vi "ActorNR.vi"(10 "Startup Message":refnum<class "MSG.lvclass">, 11 "Actor Type":refnum<class "Messenger.lvclass">) -> ()   [LabVIEW 2016, in "Messenger.lvclass"]
uses:
  Messenger.lvclass
  <vilib>/drjdpowell/Messenging/Core Messages/Message/MSG.lvclass
  <vilib>/drjdpowell/Messenging/ObserverRegister/ObserverRegistry.lvclass/ObserverRegistry.ctl
  <vilib>/drjdpowell/Messenging/Core Messages/Message/MSG.lvclass/MSG.ctl
  <vilib>/drjdpowell/Messenging/Core Messages/ErrorMessage/ErrorMSG.lvclass/ErrorMSG.ctl
  <vilib>/Utility/error.llb/DialogType.ctl
  <vilib>/drjdpowell/Messenging/Core Messages/ErrorMessage/Write ErrorMessage.vi
  <vilib>/drjdpowell/Messenging/Core Messages/MSG Library/Reply (message).vi
  <vilib>/drjdpowell/Messenging/Core Messages/MSG Library/Reply (no data).vi
  <vilib>/drjdpowell/Messenging/Core Messages/Message/Label Message.vi
  <vilib>/drjdpowell/Messenging/ObserverRegister/Read DVR.vi
  <vilib>/drjdpowell/Messenging/Core Messages/Message/Write (no data).vi
  <vilib>/drjdpowell/Messenging/Core Messages/Message/Overwrite Reply Address.vi
  <vilib>/drjdpowell/Messenging/Core Messages/ErrorMessage/ErrorMSG.lvclass
  C:/Program Files (x86)/National Instruments/LabVIEW 2016/vi.lib/drjdpowell/Messenging/Core Messages/Message/MSG.lvclass
  <vilib>/drjdpowell/Messenging/ObserverRegister/ObsReg Core/Event Notification.vi
  <vilib>/drjdpowell/Messenging/ObserverRegister/Commands/ParentCommand/ObserverRegistryCommand.lvclass
  <vilib>/drjdpowell/Messenging/Core Messengers/Send/Send.lvclass
  <vilib>/drjdpowell/Messenging/Core Messengers/EventMessenger/EventMessenger.lvclass
  <vilib>/drjdpowell/Messenging/Core Messages/MSG Library/SendMSG.lvlib
  <vilib>/drjdpowell/Messenging/ObserverRegister/ObsReg.lvlib
  <vilib>/drjdpowell/Messenging/Parallel Process/Parallel Process Library/Parallel Process.lvlib
  <vilib>/drjdpowell/Messenging/ObserverRegister/ObserverRegistry.lvclass
panel:
  # "You can make this actor shared-reentrant (many instances)\nor non-reentrant (only one instance).\nTo do so you must also rename this VI:\n     shared reentrant: \"Actor.vi\"\n     non-reentrant: \"ActorNR.vi\""
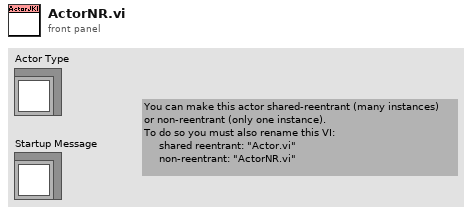
[diagram p1: front panel]
types:
  T1 = typedef "Parallel Process.lvlib/Actor Communication.ctl" = cluster{"Messenger":refnum<class "EventMessenger.lvclass">, "Private Messenger":refnum<class "EventMessenger.lvclass">, "ObsReg":refnum<class "ObserverRegistry.lvclass">, "Reg":refnum<event-registration>}
  T2 = enum32{"invalid app kind", "Development System", "Run Time System", "Student Edition", "Embedded LabVIEW", "Evaluation", "Custom"}
  T3 = enum32{"Invalid", "Standard", "Closed", "Hidden", "Minimized", "Maximized"}
  T4 = cluster{"Core":cluster{"Current VI Reference":refnum<vi>, "Close Panel on Exit?":bool, "Running Top Level":bool}, "Actor":T1, "Your Boolean data":bool, "TimeFormat":string}
  T5 = typedef "DialogType.ctl" = u16
  T6 = enum16{"Left Button", "Center Button", "Right Button", "Window Close"}
  T7 = cluster{"Current VI Reference":refnum<vi>, "Close Panel on Exit?":bool, "Running Top Level":bool}
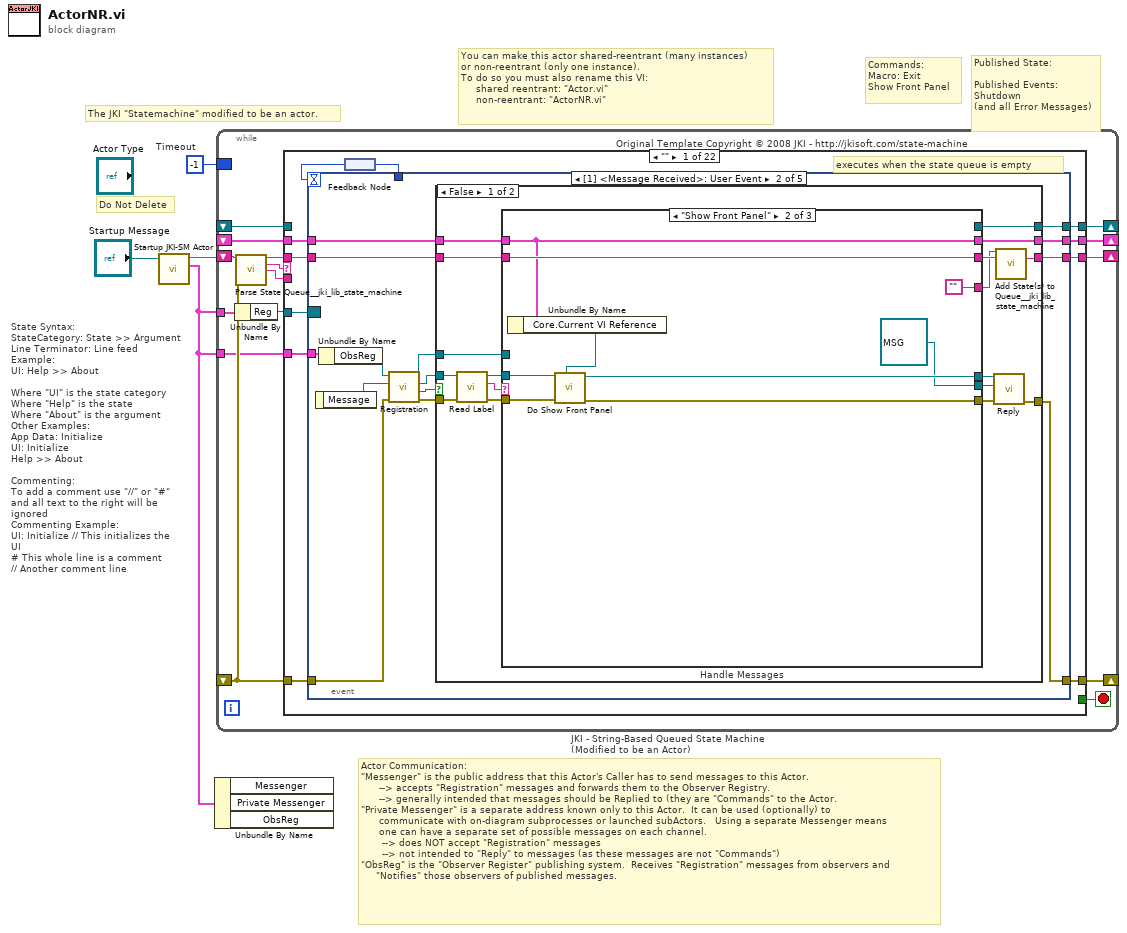
[diagram p0: block diagram]
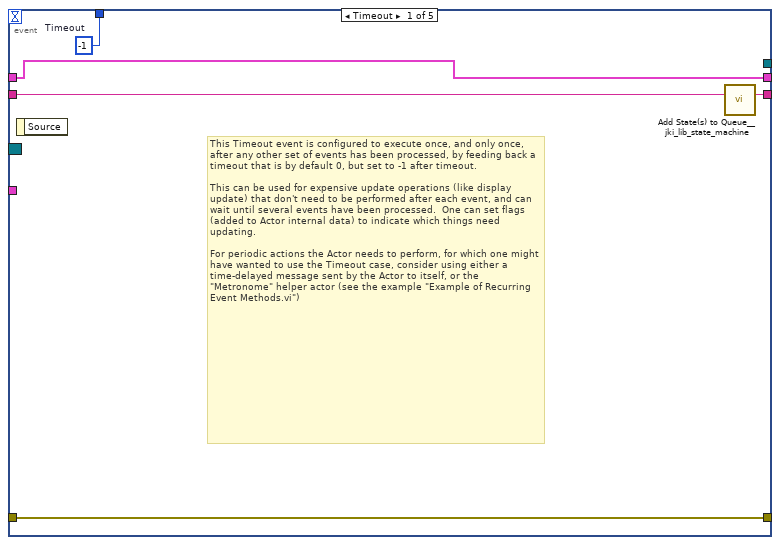
[diagram p2: hidden frame]
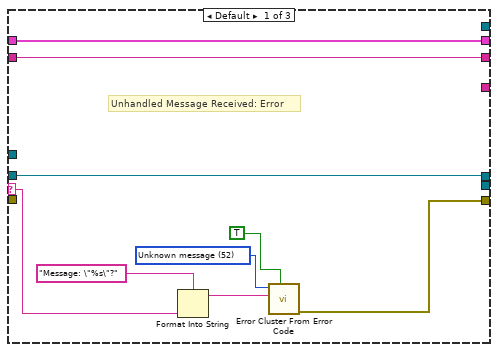
[diagram p3: hidden frame]
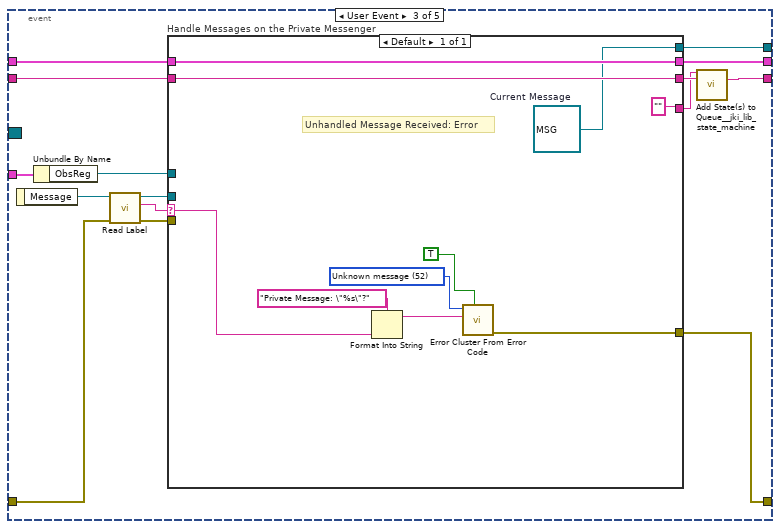
[diagram p6: hidden frame]
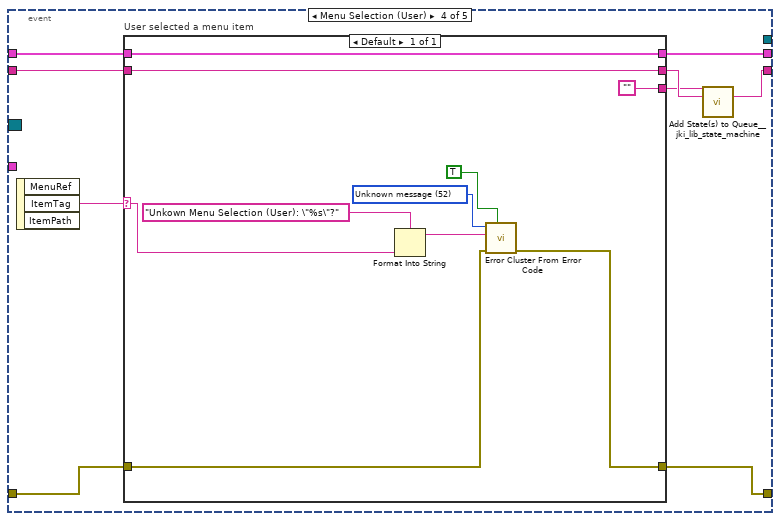
[diagram p7: hidden frame]
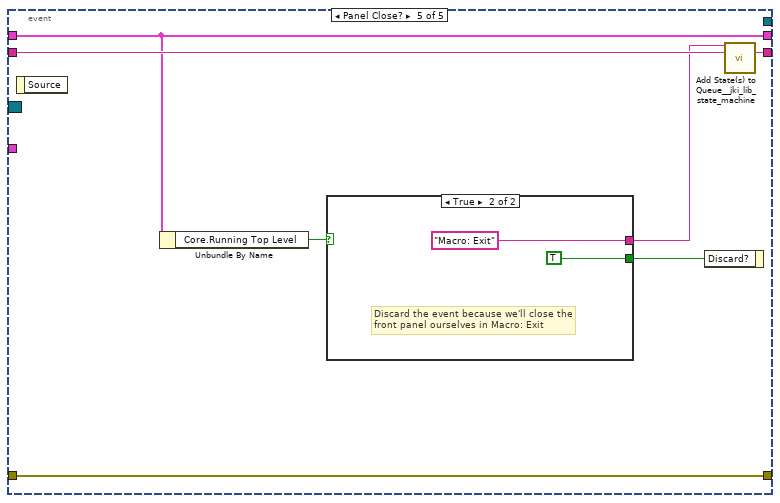
[diagram p8: hidden frame]
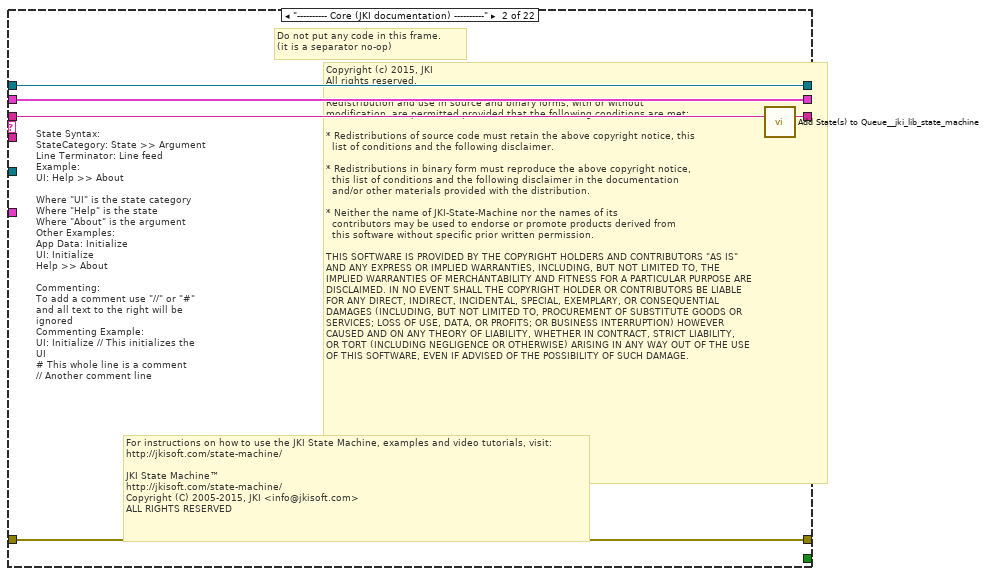
[diagram p10: hidden frame]
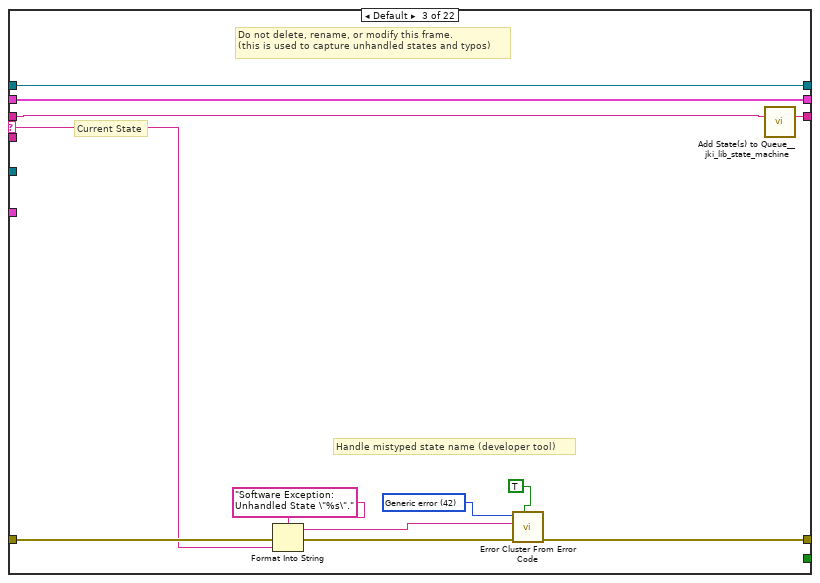
[diagram p11: hidden frame]
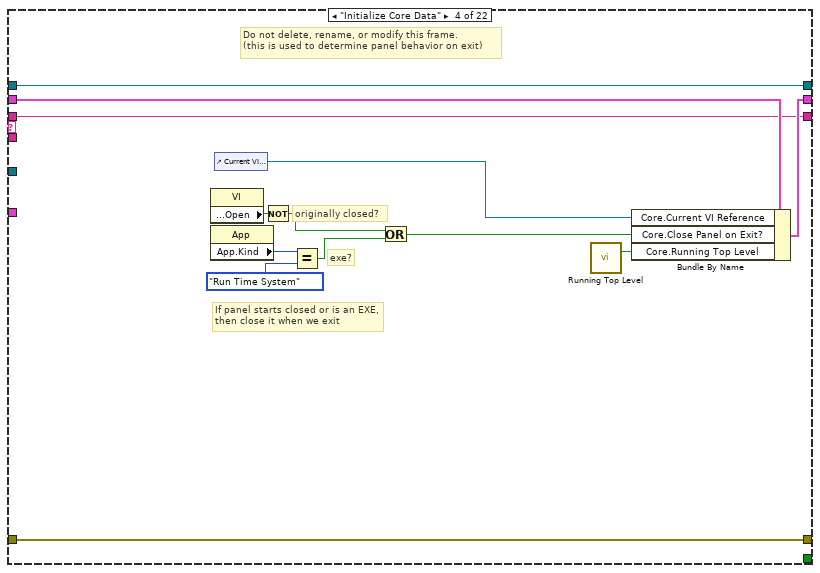
[diagram p12: hidden frame]
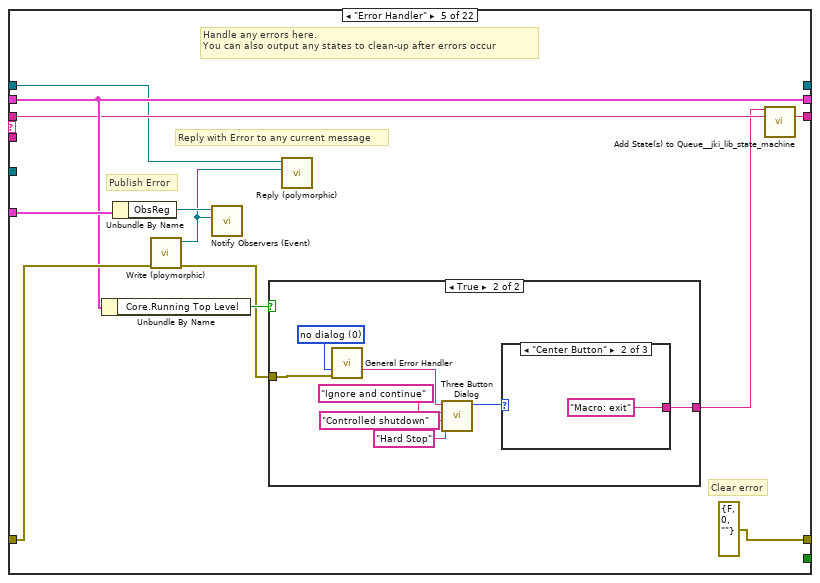
[diagram p13: hidden frame]
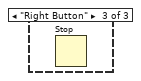
[diagram p16: hidden frame]
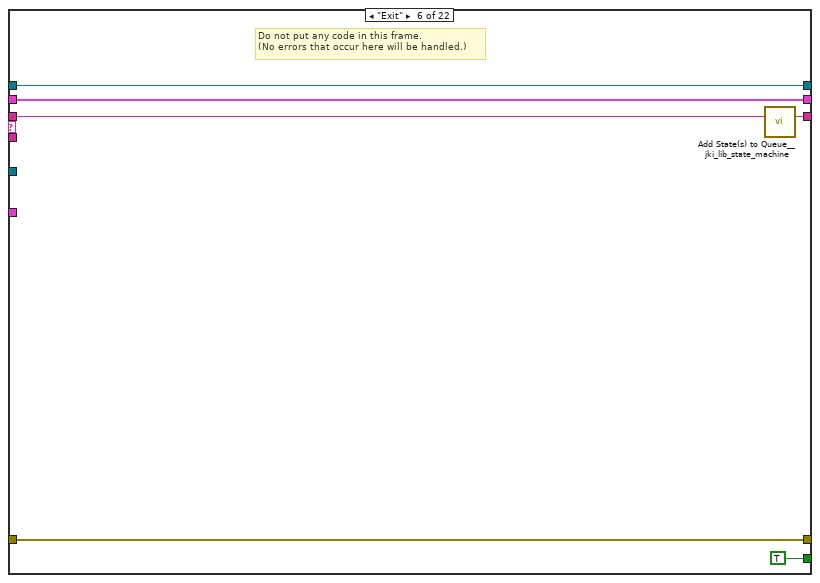
[diagram p17: hidden frame]
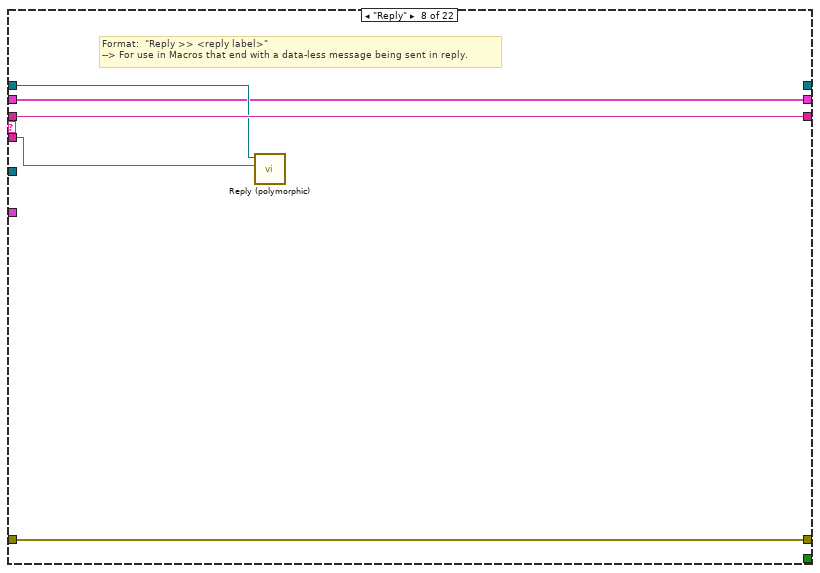
[diagram p19: hidden frame]
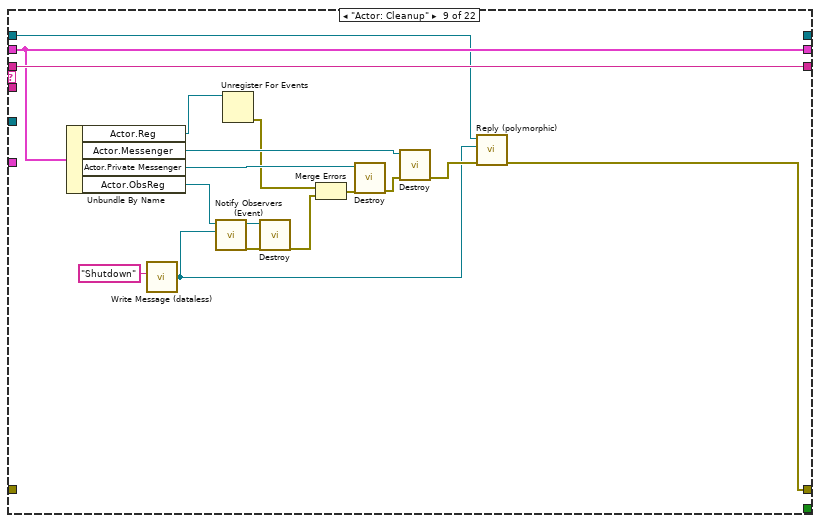
[diagram p20: hidden frame]
diagram:
  w1 = -1  # Timeout
  # "You can make this actor shared-reentrant (many instances)\nor non-reentrant (only one instance).\nTo do so you must also rename this VI:\n     shared reentrant: \"Actor.vi\"\n     non-reentrant: \"ActorNR.vi\""
  # "State Syntax:\nStateCategory: State >> Argument\nLine Terminator: Line feed\nExample:\nUI: Help >> About\n\nWhere \"UI\" is the state category\nWhere \"Help\" is the state\nWhere \"About\" is the argument\nOther Examples:\nApp Data: Initialize\nUI: Initialize\nHelp >> About\n\nCommenting:\nTo add a comment use \"//\" or \"#\" and all text to the right will be ignored\nCommenting Example:\nUI: Initialize // This initializes the UI\n# This whole line is a comment\n// Another comment line"
  # "The JKI \"Statemachine\" modified to be an actor."
  # "Actor Communication:\n\"Messenger\" is the public address that this Actor's Caller has to send messages to this Actor.\n      --> accepts \"Registration\" messages and forwards them to the Observer Registry.\n      --> generally intended that messages should be Replied to (they are \"Commands\" to the Actor.\n\"Private Messenger\" is a separate address known only to this Actor.  It can be used (optionally) to \n      communicate with on-diagram subprocesses or launched subActors.   Using a separate Messenger means\n      one can have a separate set of possible messages on each channel. \n       --> does NOT accept \"Registration\" messages\n       --> not intended to \"Reply\" to messages (as these messages are not \"Commands\")\n\"ObsReg\" is the \"Observer Register\" publishing system.  Receives \"Registration\" messages from observers and \n     \"Notifies\" those observers of published messages."
  # "Do Not Delete"
  # "Published State:\n \nPublished Events:\nShutdown\n(and all Error Messages)"
  # "Commands:\nMacro: Exit\nShow Front Panel"
  n1 = call <vilib>:"Startup JKI-SM Actor.vi"("MSG in"="Startup Message") -> ("Actor"=w2:T1, "Initial States (\"Macro: Initialize\")"=w3:string)  [unwired: 9 in]
  n2 = Unbundle By Name(w2) -> ()  [unwired: 3 out]
  n3 = while "JKI - String-Based Queued State Machine (Modified to be an Actor)" {
    shift-right: [w12] -> _
    shift-left: _ -> [w11]
    shift-right: [w15] -> _
    shift-left: _ -> [w10]
    shift-right: [w14] -> _
    shift-left: w3 -> [w16]
    tunnel: w2 -> [w7]
    tunnel: w2 -> [w9]
    shift-right: [w6] -> _
    shift-left: _ -> [w5]
    border: w1 -> [_]
    stop <- w13 stop-if-true
    # "Original Template Copyright © 2008 JKI - http://jkisoft.com/state-machine"
    n4 = Unbundle By Name(w7) -> ("Reg"=w8:refnum<event-registration>)
    n5 = call <vilib>:"Parse State Queue__jki_lib_state_machine.vi"("State Queue"=w16, "Error In (no error)"=w10) -> ("Remaining States"=w18:string, "Current State"=w19:string, "Arguments"=w17:string)  [unwired: 11 in]
    n6 = case shown="\"\"" w19 {
      selector: w19 -> [_ _ w152 _ _ _ _ _ _ _ _ _ _ _ _ _ _ _ _ _ _ _]
      tunnel: w18 -> [w30 w150 w156 w165 w182 w202 w205 w210 w221 w233 w242 w244 w253 w255 w259 w269 w298 w306 w317 w322 w327 w332]
      tunnel: w17 -> [_ _ _ _ _ _ _ w209 _ _ _ _ _ _ w260 w270 _ _ _ _ _ _]
      tunnel: w11 -> [w28 w147 w154 w168 w183 w200 w206 w207 w220 w230 _ w245 w250 w257 w263 w272 w299 w303 w314 w319 w324 w329]
      tunnel: [w27 w148 w158 w174 errorcluster {"status"=FALSE, "code"=0, "source"=""} ("error out") w199 w204 w211 w219 w231 w239 w246 w251 w256 w261 w273 w300 w304 w315 w320 w325 w330] -> w15
      tunnel: w10 -> [w26 w148 w157 w174 w185 w199 w204 w211 _ w231 w239 w247 w251 w256 w262 w274 w300 w304 w315 w320 w325 w330]
      tunnel: [w29 w149 w155 w165 w187 w201 w205 w210 w221 w232 w241 w244 w252 w255 w259 w269 w298 w305 w316 w321 w326 w331] -> w14
      tunnel: [_ _ _ _ _ TRUE _ _ _ _ _ _ _ _ _ _ _ _ _ _ _ _] -> w13
      tunnel: [w25 w147 w154 w175 w183 w200 w206 w207 w220 w230 w240 w245 w250 w257 w263 w272 w299 w303 w314 w319 w324 w329] -> w12
      tunnel: w8 -> [w24 _ _ _ _ _ _ _ _ _ _ _ _ _ _ _ _ _ _ _ _ _]
      tunnel: w9 -> [w23 _ _ _ w184 _ _ _ _ _ w236 _ _ _ _ _ _ _ _ _ _ _]
      tunnel: [w22 w146 w151 w164 _ w197 w203 _ _ w229 w234 w243 w249 w254 w258 w268 w297 w301 w307 w318 w323 w328] -> w6
      tunnel: w5 -> [_ w146 w151 w164 w181 w197 w203 w208 w214 w229 _ w243 w249 w254 w258 w268 w297 w301 w307 w318 w323 w328]
      frame "" {
        # "executes when the state queue is empty"
        n7 = feedback #1() -> (w21:i32)
        n8 = event shown="[1] <Message Received>: User Event" {
          selector: w24 -> [_ _ _ _ _]
          dyn-events: _ -> [_ _ _ _ _]
          timeout: w21 -> [_ _ _ _ _]
          tunnel: w30 -> [w35 w40 w105 w123 w143]
          tunnel: [w34 w39 w104 w119 w142] -> w29
          tunnel: w28 -> [w32 w42 w107 w124 w137]
          tunnel: [w33 w38 w94 w121 w141] -> w27
          tunnel: w26 -> [w33 w46 w103 w122 w141]
          tunnel: [w32 w41 w106 w125 w137] -> w25
          tunnel: w23 -> [_ w49 w101 _ _]
          tunnel: [_ w36 w93 _ _] -> w22
          tunnel: [w31 _ _ _ _] -> w20
          event Timeout {
            w31 = -1  # Timeout
            # "This Timeout event is configured to execute once, and only once, after any other set of events has been processed, by feeding back a timeout that is by default 0, but set to -1 after timeout.  \n\nThis can be used for expensive update operations (like display update) that don't need to be performed after each event, and can wait until several events have been processed.  One can set flags (added to Actor internal data) to indicate which things need updating.\n\nFor periodic actions the Actor needs to perform, for which one might have wanted to use the Timeout case, consider using either a time-delayed message sent by the Actor to itself, or the \"Metronome\" helper actor (see the example \"Example of Recurring Event Methods.vi\")"
            n9 = event-data() -> ()  [unwired: 1 in, 1 out]
            n10 = call <vilib>:"Add State(s) to Queue__jki_lib_state_machine.vi"("State(s) in (\"\")"=w35) -> ("States Out"=w34:string)  [unwired: 14 in]
          }
          event User Event {
            n11 = event-data() -> ("Message"=w47:refnum<class "MSG.lvclass">)  [unwired: 1 in]
            n12 = Unbundle By Name(w49) -> ("ObsReg"=w48:refnum<class "ObserverRegistry.lvclass">)
            n13 = call <vilib>:"Registration.vi"("error in (no error)"=w46, "Message"=w47, "Observer Registry"=w48) -> ("error out"=w43:errorcluster, "Message Was a Registration Message"=w45:bool, "Message (Registration messages filtered out)"=w44:refnum<class "MSG.lvclass">, "Observer Registry"=w37:refnum<class "ObserverRegistry.lvclass">)  [unwired: 5 in]
            n14 = case shown="False" w45 {
              tunnel: w44 -> [w66 _]
              tunnel: w43 -> [w65 w90]
              tunnel: w42 -> [w61 w92]
              tunnel: [w60 w92] -> w41
              tunnel: w40 -> [w59 w91]
              tunnel: [w57 w91] -> w39
              tunnel: [w53 w90] -> w38
              tunnel: w37 -> [w51 _]
              tunnel: [w50 _] -> w36
              frame False {
                n15 = call-dynamic "Read Label.vi"("error in (no error)"=w65, "Message"=w66) -> ("error out"=w62:errorcluster, "Label"=w64:string, "Message"=w63:refnum<class "MSG.lvclass">)  [unwired: 7 in]
                n16 = case "Handle Messages" shown="\"Show Front Panel\"" w64 {
                  selector: w64 -> [w68 _ w87]
                  tunnel: w63 -> [w73 w83 w86]
                  tunnel: w62 -> [_ w82 w88]
                  tunnel: w61 -> [w74 w77 w85]
                  tunnel: [w74 w77 w85] -> w60
                  tunnel: w59 -> [w75 w84 w89]
                  tunnel: [w75 w84 w89] -> w58
                  tunnel: [_ "" w87] -> w56
                  tunnel: [w73 w81 _] -> w55
                  tunnel: [w67 w80 w88] -> w54
                  tunnel: [_ refnum<class "MSG.lvclass"> refnum ("Message (data extracted)") _] -> w52
                  tunnel: w51 -> [_ _ _]
                  tunnel: [_ _ w86] -> w50
                  frame Default {
                    w71 = 52 items=["No error", "Argument error", "Memory is full", "Out of zone", "End of file", "File already open", "Generic file I/O error", "File not found", "File permission error", "Disk is full", "Duplicate path", "Too many files open", "System feature not enabled", "Resource file not found", "Cannot add resource", "Resource not found", "Image not found", "Image memory error", "Pen does not exist", "Config type invalid", "Config token not found", "Config parse error", "Config memory error", "Bad external code format", "Bad external code offset", "External code not present", "Null window", "Destroy window error", "Null menu", "Print aborted", "Bad print record", "Print driver error", "Windows error during printing", "Memory error during printing", "Print dialog error", "Generic print error", "Invalid device refnum", "Device not found", "Device parameter error", "Device unit error", "Cannot open device", "Device call aborted", "Generic error", "Cancelled by user", "Object ID too low", "Object ID too high", "Object not in heap", "Unknown heap", "Unknown object (invalid DefProc)", "Unknown object (DefProc not in table)", "Message out of range", "Invalid (null) method", "Unknown message", "Manager call not supported", "Bad address", "Network operation in progress", "Network operation timed out", "Connection is busy", "Network attribute not supported", "Network error", "Address in use", "System out of memory", "Connection aborted", "Connection refused", "Not connected", "Already connected", "Connection closed", "Initialization error (interapplication manager)", "Bad occurrence", "Wait on unbound occurrence handler", "Occurrence queue overflow", "Datalog type conflict", "Unused", "Unrecognized type (interapplication manager)", "Memory corrupt", "Failed to make temporary DLL", "Old CIN version", "Drag socket not found", "Failed to load drop-object", "Failed to register OLE object", "Failed to release OLE object", "Format specifier type mismatch", "Unknown format specifier", "Too few format specifiers", "Too many format specifiers", "Scan failed", "Newer CIN version", "Error converting to variant", "Runtime menu error", "Password tampered", "Variant attribute not found", "Incompatible variant data type", "Event data is not available", "Event Store is not present", "Occurrence is not found", "Event Queue is not created", "Event info is not available", "Refnum passed is NULL", "Error retrieving Class GUID", "Error retrieving CoClass GUID", "Error retrieving TypeLib GUID.", "Bad built application magic bytes.", "Specific driver is different from the specific driver associated with the Logical Name.", "There is no session opened to the class driver.", "Max Error", "MAX - Error with config objects", "MAX - Error loading configuration", "MAX - Group not supported"]
                    # "Unhandled Message Received: Error"
                    n17 = Format Into String(format string="Message: \"%s\"?", w68) -> (resulting string=w70:string)  [unwired: 2 in, 1 out]
                    n18 = call <vilib>:"Error Cluster From Error Code.vi"("show call chain? (False)"=TRUE, "error message (\"\")"=w70, "error code (0)"=w71) -> ("error out"=w67:errorcluster)  [unwired: 1 in, 5 out]
                  }
                  frame "Show Front Panel" {
                    n19 = Unbundle By Name(w77) -> ("Core.Current VI Reference"=w76:refnum<vi>)
                    n20 = call <vilib>:"Do Show Front Panel.vi"("Front Panel (Calling VI)"=w76, "error in (no error)"=w82, "MSG in"=w83) -> ("error out"=w80:errorcluster, "Message (data extracted)"=w81:refnum<class "MSG.lvclass">)  [unwired: 7 in]
                  }
                  frame "Macro: Exit" {
                  }
                }
                n21 = call <vilib>:"Reply.vi"("error in (no error)"=w54, "Reply"=w52, "Message to Reply to"=w55) -> ("error out"=w53:errorcluster)  [unwired: 7 in, 1 out]
                n22 = call <vilib>:"Add State(s) to Queue__jki_lib_state_machine.vi"("State(s) in Front (\"\")"=w56, "State(s) in (\"\")"=w58) -> ("States Out"=w57:string)  [unwired: 13 in]
              }
              frame True {
                # "Message was  for the Observer Registry and has been processed."
              }
            }
          }
          event User Event {
            n23 = event-data() -> ("Message"=w102:refnum<class "MSG.lvclass">)  [unwired: 1 in]
            n24 = Unbundle By Name(w101) -> ("ObsReg"=w100:refnum<class "ObserverRegistry.lvclass">)
            n25 = call-dynamic "Read Label.vi"("error in (no error)"=w103, "Message"=w102) -> ("error out"=w97:errorcluster, "Label"=w99:string, "Message"=w98:refnum<class "MSG.lvclass">)  [unwired: 7 in]
            n26 = case "Handle Messages on the Private Messenger" shown="Default" w99 {
              selector: w99 -> [w111]
              tunnel: w98 -> [_]
              tunnel: w97 -> [_]
              tunnel: w107 -> [w116]
              tunnel: [w116] -> w106
              tunnel: w105 -> [w117]
              tunnel: [w117] -> w96
              tunnel: [""] -> w95
              tunnel: w100 -> [_]
              tunnel: [w109] -> w94
              tunnel: [w108] -> w93
              frame Default {
                w108 = refnum<class "MSG.lvclass"> refnum  # Current Message
                w114 = 52 items=["No error", "Argument error", "Memory is full", "Out of zone", "End of file", "File already open", "Generic file I/O error", "File not found", "File permission error", "Disk is full", "Duplicate path", "Too many files open", "System feature not enabled", "Resource file not found", "Cannot add resource", "Resource not found", "Image not found", "Image memory error", "Pen does not exist", "Config type invalid", "Config token not found", "Config parse error", "Config memory error", "Bad external code format", "Bad external code offset", "External code not present", "Null window", "Destroy window error", "Null menu", "Print aborted", "Bad print record", "Print driver error", "Windows error during printing", "Memory error during printing", "Print dialog error", "Generic print error", "Invalid device refnum", "Device not found", "Device parameter error", "Device unit error", "Cannot open device", "Device call aborted", "Generic error", "Cancelled by user", "Object ID too low", "Object ID too high", "Object not in heap", "Unknown heap", "Unknown object (invalid DefProc)", "Unknown object (DefProc not in table)", "Message out of range", "Invalid (null) method", "Unknown message", "Manager call not supported", "Bad address", "Network operation in progress", "Network operation timed out", "Connection is busy", "Network attribute not supported", "Network error", "Address in use", "System out of memory", "Connection aborted", "Connection refused", "Not connected", "Already connected", "Connection closed", "Initialization error (interapplication manager)", "Bad occurrence", "Wait on unbound occurrence handler", "Occurrence queue overflow", "Datalog type conflict", "Unused", "Unrecognized type (interapplication manager)", "Memory corrupt", "Failed to make temporary DLL", "Old CIN version", "Drag socket not found", "Failed to load drop-object", "Failed to register OLE object", "Failed to release OLE object", "Format specifier type mismatch", "Unknown format specifier", "Too few format specifiers", "Too many format specifiers", "Scan failed", "Newer CIN version", "Error converting to variant", "Runtime menu error", "Password tampered", "Variant attribute not found", "Incompatible variant data type", "Event data is not available", "Event Store is not present", "Occurrence is not found", "Event Queue is not created", "Event info is not available", "Refnum passed is NULL", "Error retrieving Class GUID", "Error retrieving CoClass GUID", "Error retrieving TypeLib GUID.", "Bad built application magic bytes.", "Specific driver is different from the specific driver associated with the Logical Name.", "There is no session opened to the class driver.", "Max Error", "MAX - Error with config objects", "MAX - Error loading configuration", "MAX - Group not supported"]
                # "Unhandled Message Received: Error"
                n27 = Format Into String(format string="Private Message: \"%s\"?", w111) -> (resulting string=w113:string)  [unwired: 2 in, 1 out]
                n28 = call <vilib>:"Error Cluster From Error Code.vi"("show call chain? (False)"=TRUE, "error message (\"\")"=w113, "error code (0)"=w114) -> ("error out"=w109:errorcluster)  [unwired: 1 in, 5 out]
              }
            }
            n29 = call <vilib>:"Add State(s) to Queue__jki_lib_state_machine.vi"("State(s) in Front (\"\")"=w95, "State(s) in (\"\")"=w96) -> ("States Out"=w104:string)  [unwired: 13 in]
          }
          event Menu Selection (User) {
            n30 = event-data() -> ("ItemTag"=w126:string)  [unwired: 1 in, 2 out]
            n31 = case "User selected a menu item" shown="Default" w126 {
              selector: w126 -> [w130]
              tunnel: [w136] -> w125
              tunnel: w124 -> [w136]
              tunnel: [w135] -> w120
              tunnel: w123 -> [w135]
              tunnel: w122 -> [w128]
              tunnel: [w129] -> w121
              tunnel: [""] -> w118
              frame Default {
                w133 = 52 items=["No error", "Argument error", "Memory is full", "Out of zone", "End of file", "File already open", "Generic file I/O error", "File not found", "File permission error", "Disk is full", "Duplicate path", "Too many files open", "System feature not enabled", "Resource file not found", "Cannot add resource", "Resource not found", "Image not found", "Image memory error", "Pen does not exist", "Config type invalid", "Config token not found", "Config parse error", "Config memory error", "Bad external code format", "Bad external code offset", "External code not present", "Null window", "Destroy window error", "Null menu", "Print aborted", "Bad print record", "Print driver error", "Windows error during printing", "Memory error during printing", "Print dialog error", "Generic print error", "Invalid device refnum", "Device not found", "Device parameter error", "Device unit error", "Cannot open device", "Device call aborted", "Generic error", "Cancelled by user", "Object ID too low", "Object ID too high", "Object not in heap", "Unknown heap", "Unknown object (invalid DefProc)", "Unknown object (DefProc not in table)", "Message out of range", "Invalid (null) method", "Unknown message", "Manager call not supported", "Bad address", "Network operation in progress", "Network operation timed out", "Connection is busy", "Network attribute not supported", "Network error", "Address in use", "System out of memory", "Connection aborted", "Connection refused", "Not connected", "Already connected", "Connection closed", "Initialization error (interapplication manager)", "Bad occurrence", "Wait on unbound occurrence handler", "Occurrence queue overflow", "Datalog type conflict", "Unused", "Unrecognized type (interapplication manager)", "Memory corrupt", "Failed to make temporary DLL", "Old CIN version", "Drag socket not found", "Failed to load drop-object", "Failed to register OLE object", "Failed to release OLE object", "Format specifier type mismatch", "Unknown format specifier", "Too few format specifiers", "Too many format specifiers", "Scan failed", "Newer CIN version", "Error converting to variant", "Runtime menu error", "Password tampered", "Variant attribute not found", "Incompatible variant data type", "Event data is not available", "Event Store is not present", "Occurrence is not found", "Event Queue is not created", "Event info is not available", "Refnum passed is NULL", "Error retrieving Class GUID", "Error retrieving CoClass GUID", "Error retrieving TypeLib GUID.", "Bad built application magic bytes.", "Specific driver is different from the specific driver associated with the Logical Name.", "There is no session opened to the class driver.", "Max Error", "MAX - Error with config objects", "MAX - Error loading configuration", "MAX - Group not supported"]
                n32 = Format Into String(format string="Unkown Menu Selection (User): \"%s\"?", w130) -> (resulting string=w132:string)  [unwired: 2 in, 1 out]
                n33 = call <vilib>:"Error Cluster From Error Code.vi"("show call chain? (False)"=TRUE, "error in (no error)"=w128, "error message (\"\")"=w132, "error code (0)"=w133) -> ("error out"=w129:errorcluster)  [unwired: 5 out]
              }
            }
            n34 = call <vilib>:"Add State(s) to Queue__jki_lib_state_machine.vi"("State(s) in Front (\"\")"=w118, "State(s) in (\"\")"=w120) -> ("States Out"=w119:string)  [unwired: 13 in]
          }
          event Panel Close? {
            n35 = event-data() -> ()  [unwired: 1 in, 1 out]
            n36 = Unbundle By Name(w137) -> ("Core.Running Top Level"=w140:bool)
            n37 = case shown="True" w140 {
              tunnel: [_ "Macro: Exit"] -> w138
              tunnel: [_ TRUE ("Discard?")] -> w139
              frame False {
              }
              frame True {
                # "Discard the event because we'll close the front panel ourselves in Macro: Exit"
              }
            }
            n38 = event-data("Discard?"=w139) -> ()  [unwired: 1 in, 1 out]
            n39 = call <vilib>:"Add State(s) to Queue__jki_lib_state_machine.vi"("State(s) in Front (\"\")"=w138, "State(s) in (\"\")"=w143) -> ("States Out"=w142:string)  [unwired: 13 in]
          }
        }
        n40 = feedback-in #1(w20) -> ()
      }
      frame "---------- Core (JKI documentation) ----------" {
        # "For instructions on how to use the JKI State Machine, examples and video tutorials, visit:\nhttp://jkisoft.com/state-machine/\n\nJKI State Machine™\nhttp://jkisoft.com/state-machine/\nCopyright (C) 2005-2015, JKI <info@jkisoft.com>\nALL RIGHTS RESERVED"
        # "State Syntax:\nStateCategory: State >> Argument\nLine Terminator: Line feed\nExample:\nUI: Help >> About\n\nWhere \"UI\" is the state category\nWhere \"Help\" is the state\nWhere \"About\" is the argument\nOther Examples:\nApp Data: Initialize\nUI: Initialize\nHelp >> About\n\nCommenting:\nTo add a comment use \"//\" or \"#\" and all text to the right will be ignored\nCommenting Example:\nUI: Initialize // This initializes the UI\n# This whole line is a comment\n// Another comment line"
        # "Copyright (c) 2015, JKI\nAll rights reserved.\n\nRedistribution and use in source and binary forms, with or without\nmodification, are permitted provided that the following conditions are met:\n\n* Redistributions of source code must retain the above copyright notice, this\n  list of conditions and the following disclaimer.\n\n* Redistributions in binary form must reproduce the above copyright notice,\n  this list of conditions and the following disclaimer in the documentation\n  and/or other materials provided with the distribution.\n\n* Neither the name of JKI-State-Machine nor the names of its\n  contributors may be used to endorse or promote products derived from\n  this software without specific prior written permission.\n\nTHIS SOFTWARE IS PROVIDED BY THE COPYRIGHT HOLDERS AND CONTRIBUTORS \"AS IS\"\nAND ANY EXPRESS OR IMPLIED WARRANTIES, INCLUDING, BUT NOT LIMITED TO, THE\nIMPLIED WARRANTIES OF MERCHANTABILITY AND FITNESS FOR A PARTICULAR PURPOSE ARE\nDISCLAIMED. IN NO EVENT SHALL THE COPYRIGHT HOLDER OR CONTRIBUTORS BE LIABLE\nFOR ANY DIRECT, INDIRECT, INCIDENTAL, SPECIAL, EXEMPLARY, OR CONSEQUENTIAL\nDAMAGES (INCLUDING, BUT NOT LIMITED TO, PROCUREMENT OF SUBSTITUTE GOODS OR\nSERVICES; LOSS OF USE, DATA, OR PROFITS; OR BUSINESS INTERRUPTION) HOWEVER\nCAUSED AND ON ANY THEORY OF LIABILITY, WHETHER IN CONTRACT, STRICT LIABILITY,\nOR TORT (INCLUDING NEGLIGENCE OR OTHERWISE) ARISING IN ANY WAY OUT OF THE USE\nOF THIS SOFTWARE, EVEN IF ADVISED OF THE POSSIBILITY OF SUCH DAMAGE."
        # "Do not put any code in this frame.\n(it is a separator no-op)"
        n41 = call <vilib>:"Add State(s) to Queue__jki_lib_state_machine.vi"("State(s) in (\"\")"=w150) -> ("States Out"=w149:string)  [unwired: 14 in]
      }
      frame Default {
        w161 = 42 items=["No error", "Argument error", "Memory is full", "Out of zone", "End of file", "File already open", "Generic file I/O error", "File not found", "File permission error", "Disk is full", "Duplicate path", "Too many files open", "System feature not enabled", "Resource file not found", "Cannot add resource", "Resource not found", "Image not found", "Image memory error", "Pen does not exist", "Config type invalid", "Config token not found", "Config parse error", "Config memory error", "Bad external code format", "Bad external code offset", "External code not present", "Null window", "Destroy window error", "Null menu", "Print aborted", "Bad print record", "Print driver error", "Windows error during printing", "Memory error during printing", "Print dialog error", "Generic print error", "Invalid device refnum", "Device not found", "Device parameter error", "Device unit error", "Cannot open device", "Device call aborted", "Generic error", "Cancelled by user", "Object ID too low", "Object ID too high", "Object not in heap", "Unknown heap", "Unknown object (invalid DefProc)", "Unknown object (DefProc not in table)", "Message out of range", "Invalid (null) method", "Unknown message", "Manager call not supported", "Bad address", "Network operation in progress", "Network operation timed out", "Connection is busy", "Network attribute not supported", "Network error", "Address in use", "System out of memory", "Connection aborted", "Connection refused", "Not connected", "Already connected", "Connection closed", "Initialization error (interapplication manager)", "Bad occurrence", "Wait on unbound occurrence handler", "Occurrence queue overflow", "Datalog type conflict", "Unused", "Unrecognized type (interapplication manager)", "Memory corrupt", "Failed to make temporary DLL", "Old CIN version", "Drag socket not found", "Failed to load drop-object", "Failed to register OLE object", "Failed to release OLE object", "Format specifier type mismatch", "Unknown format specifier", "Too few format specifiers", "Too many format specifiers", "Scan failed", "Newer CIN version", "Error converting to variant", "Runtime menu error", "Password tampered", "Variant attribute not found", "Incompatible variant data type", "Event data is not available", "Event Store is not present", "Occurrence is not found", "Event Queue is not created", "Event info is not available", "Refnum passed is NULL", "Error retrieving Class GUID", "Error retrieving CoClass GUID", "Error retrieving TypeLib GUID.", "Bad built application magic bytes.", "Specific driver is different from the specific driver associated with the Logical Name.", "There is no session opened to the class driver.", "Max Error", "MAX - Error with config objects", "MAX - Error loading configuration", "MAX - Group not supported"]
        # "Current State"
        # "Do not delete, rename, or modify this frame.\n(this is used to capture unhandled states and typos)"
        # "Handle mistyped state name (developer tool)"
        n42 = Format Into String(format string="Software Exception: Unhandled State \"%s\"." ("message"), error in=w157, w152) -> (resulting string=w160:string, error out=w159:errorcluster)  [unwired: 1 in]
        n43 = call <vilib>:"Error Cluster From Error Code.vi"("show call chain? (False)"=TRUE, "error in (no error)"=w159, "error message (\"\")"=w160, "error code (0)"=w161) -> ("error out"=w158:errorcluster)  [unwired: 5 in]
        n44 = call <vilib>:"Add State(s) to Queue__jki_lib_state_machine.vi"("State(s) in (\"\")"=w156) -> ("States Out"=w155:string)  [unwired: 14 in]
      }
      frame "Initialize Core Data" {
        # "Do not delete, rename, or modify this frame.\n(this is used to determine panel behavior on exit)"
        # "originally closed?"
        # "exe?"
        # "If panel starts closed or is an EXE, then close it when we exit"
        n45 = property class="VI"() -> ("Front Panel.Open"=w173:bool)  [unwired: 2 in, 2 out]
        n46 = property class="App"() -> ("App.Kind"=w172:T2)  [unwired: 2 in, 2 out]
        n47 = control-ref of="Current VI Reference"() -> (w166:refnum<vi>)
        n48 = Not(x=w173) -> (.not. x?=w170:bool)
        n49 = Equal?(x=w172, y=T2."Run Time System" ("Application:Kind")) -> (x = y?=w169:bool)
        n50 = Or(x=w170, y=w169) -> (x .or. y?=w167:bool)
        n51 = call <vilib>:"Running Top Level.vi"() -> ("Running Top Level"=w163:bool)  [unwired: 11 in]
        n52 = Bundle By Name(cluster=w168, "Core.Current VI Reference"=w166, "Core.Close Panel on Exit?"=w167, "Core.Running Top Level"=w163) -> (w175:T4)
      }
      frame "Error Handler" {
        # "Reply with Error to any current message"
        # "Publish Error"
        # "Handle any errors here.\nYou can also output any states to clean-up after errors occur"
        # "Clear error"
        n53 = Unbundle By Name(w183) -> ("Core.Running Top Level"=w178:bool)
        n54 = Unbundle By Name(w184) -> ("ObsReg"=w180:refnum<class "ObserverRegistry.lvclass">)
        n55 = call-poly <vilib>:"Write (ploymorphic).vi"("error (to be sent)"=w185) -> ("error out"=w177:errorcluster, "Message"=w179:refnum<class "ErrorMSG.lvclass">)  [unwired: 9 in]
        n56 = call <vilib>:"Notify Observers (Event).vi"("Message"=w179, "Observer Registry"=w180) -> ()  [unwired: 1 in, 9 out]
        n57 = case shown="True" w178 {
          tunnel: w177 -> [_ w195]
          tunnel: [_ w194] -> w176
          frame False {
          }
          frame True {
            w193 = T5 0 items=["no dialog", "OK message", "continue or stop message", "OK message + warnings", "continue/stop + warnings"] ("type of dialog (OK msg:1)")
            n58 = call <vilib>:"General Error Handler.vi"("type of dialog (OK msg:1)"=w193, "error in (no error)"=w195) -> ("message"=w192:string)  [unwired: 9 in, 4 out]
            n59 = call <vilib>:"Three Button Dialog.vi"("Right Button Text (\"Cancel\")"="Hard Stop" ("Right Button Text (\"Cancel\")"), "Center Button Text (\"No\")"="Controlled shutdown" ("Center Button Text (\"No\")"), "Left Button Text (\"Yes\")"="Ignore and continue" ("Left Button Text (\"Yes\")"), "message"=w192) -> ("Which Button?"=w188:T6)  [unwired: 7 in]
            n60 = case shown="\"Center Button\"" w188 {
              tunnel: [_ "Macro: exit" _] -> w194
              frame "Left Button", "Window Close" {
              }
              frame "Center Button" {
              }
              frame "Right Button" {
                n61 = Stop() -> ()  [unwired: 1 in]
              }
            }
          }
        }
        n62 = call-poly <vilib>:"Reply (polymorphic).vi"("Reply"=w179, "Message to Reply to"=w181) -> ()  [unwired: 8 in, 2 out]
        n63 = call <vilib>:"Add State(s) to Queue__jki_lib_state_machine.vi"("State(s) in Front (\"\")"=w176, "State(s) in (\"\")"=w182) -> ("States Out"=w187:string)  [unwired: 13 in]
      }
      frame "Exit" {
        # "Do not put any code in this frame.\n(No errors that occur here will be handled.)"
        n64 = call <vilib>:"Add State(s) to Queue__jki_lib_state_machine.vi"("State(s) in (\"\")"=w202) -> ("States Out"=w201:string)  [unwired: 14 in]
      }
      frame "------------ Actor ------------" {
      }
      frame "Reply" {
        # "Format:  \"Reply >> <reply label>\"\n--> For use in Macros that end with a data-less message being sent in reply."
        n65 = call-poly <vilib>:"Reply (polymorphic).vi"("Reply Label"=w209, "Message to Reply to"=w208) -> ()  [unwired: 8 in, 2 out]
      }
      frame "Actor: Cleanup" {
        n66 = Unbundle By Name(w220) -> ("Actor.Reg"=w218:refnum<event-registration>, "Actor.Messenger"=w223:refnum<class "EventMessenger.lvclass">, "Actor.Private Messenger"=w225:refnum<class "EventMessenger.lvclass">, "Actor.ObsReg"=w226:refnum<class "ObserverRegistry.lvclass">)
        n67 = call <vilib>:"Write Message (dataless).vi"("Label"="Shutdown" ("Prefix to add")) -> ("Message"=w212:refnum<class "MSG.lvclass">)  [unwired: 7 in]
        n68 = call <vilib>:"Notify Observers (Event).vi"("Message"=w212, "Observer Registry"=w226) -> ("error out"=w228:errorcluster, "Observer Registry"=w227:refnum<class "ObserverRegistry.lvclass">)  [unwired: 1 in, 7 out]
        n69 = Unregister For Events(event registration refnum=w218) -> (error out=w215:errorcluster)  [unwired: 1 in]
        n70 = call <vilib>:"Destroy.vi"("error in (no error)"=w228, "ObserverRegistry.lvclass in"=w227) -> ("error out"=w216:errorcluster)  [unwired: 9 in]
        n71 = Merge Errors(w215, w216) -> (w217:errorcluster)
        n72 = call-dynamic <vilib>:"Destroy.vi"("error in (no error)"=w217, "EventMessenger in"=w225) -> ("error out"=w224:errorcluster)  [unwired: 9 in]
        n73 = call-dynamic <vilib>:"Destroy.vi"("error in (no error)"=w224, "EventMessenger in"=w223) -> ("error out"=w222:errorcluster)  [unwired: 9 in]
        n74 = call-poly <vilib>:"Reply (polymorphic).vi"("error in (no error)"=w222, "Reply"=w212, "Message to Reply to"=w214) -> ("error out"=w219:errorcluster)  [unwired: 7 in, 1 out]
      }
      frame "---------- Data ----------" {
        # "Do not put any code in this frame.\n(It is a separator no-op. You can make a copy of this frame to create a new Data frame)"
        n75 = call <vilib>:"Add State(s) to Queue__jki_lib_state_machine.vi"("State(s) in (\"\")"=w233) -> ("States Out"=w232:string)  [unwired: 14 in]
      }
      frame "Data: Initialize" {
        w235 = "%c"  # TimeFormat
        w234 = refnum<class "MSG.lvclass"> refnum  # Current Message
        w237 = T7 {"Current VI Reference"=refnum, "Close Panel on Exit?"=FALSE, "Running Top Level"=FALSE}  # Core
        w238 = TRUE  # Your Boolean data
        # "do not delete - used by framework"
        # "Expand Bundle to add new data elements to shift register data."
        # "Add new data here."
        # "Data names and types of shift register data are defined by this bundle."
        # "Initialize the shift-register data, here.\n(data names are defined by what you wire into the bundle function)"
        n76 = Bundle("Core"=w237, "Actor"=w236, "Your Boolean data"=w238, "TimeFormat"=w235) -> (w240:T4)  [unwired: 1 in]
        n77 = call <vilib>:"Add State(s) to Queue__jki_lib_state_machine.vi"("State(s) in (\"\")"=w242) -> ("States Out"=w241:string)  [unwired: 14 in]
      }
      frame "Data: Cleanup" {
        # "Cleanup any data and references, here.\n(this is called automatically, by the Macro: Exit)"
        n78 = Unbundle By Name(w245) -> ("Core.Current VI Reference"=w248:refnum<vi>)
        n79 = Close Reference(reference=w248, error in (no error)=w247) -> (error out=w246:errorcluster)
      }
      frame "---------- UI ----------" {
        # "Do not put any code in this frame.\n(It is a separator no-op. You can make a copy of this frame to create a new UI frame)"
        n80 = call <vilib>:"Add State(s) to Queue__jki_lib_state_machine.vi"("State(s) in (\"\")"=w253) -> ("States Out"=w252:string)  [unwired: 14 in]
      }
      frame "UI: Initialize" {
        # "Initialize the User Interface, here.\n(this is called automatically, by the Macro: Init)"
      }
      frame "UI: Cursor Set" {
        # "Argument"
        # "Set and Unset Cursor Busy.\n(Usage: \"UI: Cursor Set >> Busy|Idle\")"
        n81 = case shown="\"Idle\", Default" w260 {
          tunnel: w262 -> [w265 w267]
          tunnel: [w264 w266] -> w261
          frame "Idle", Default {
            n82 = call <vilib>:"Unset Busy.vi"("error in (no error)"=w265) -> ("error out"=w264:errorcluster)  [unwired: 10 in]
          }
          frame "Busy" {
            n83 = call <vilib>:"Set Busy.vi"("error in (no error)"=w267) -> ("error out"=w266:errorcluster)  [unwired: 9 in, 1 out]
          }
        }
      }
      frame "UI: Front Panel State" {
        # "Argument"
        # "Set Front Panel Open or Closed\n(Usage: \"UI: Front Panel State >> Open|Close\")"
        n84 = Unbundle By Name(w272) -> ("Core.Current VI Reference"=w271:refnum<vi>)
        n85 = case shown="\"Open\", Default" w270 {
          tunnel: w274 -> [w278 w291]
          tunnel: [w280 w292] -> w273
          tunnel: w271 -> [w279 w289]
          frame "Open", Default {
            n86 = property class="VI"(reference=w279, error in=w278) -> (reference out=w276:refnum<vi>, error out=w277:errorcluster, "Front Panel.Open"=w275:bool)
            n87 = case shown="False" w275 {
              tunnel: [w283 w286] -> w280
              tunnel: w277 -> [w282 w286]
              tunnel: w276 -> [w281 _]
              frame False {
                n88 = invoke class="VI" method="FP.Open"(reference=w281, error in=w282, "Activate"=TRUE, "State"=T3."Standard") -> (error out=w283:errorcluster)  [unwired: 1 in, 4 out]
              }
              frame True {
              }
            }
          }
          frame "Close" {
            n89 = property class="VI"(reference=w289, error in=w291) -> (reference out=w288:refnum<vi>, error out=w290:errorcluster, "Front Panel.Open"=w287:bool)
            n90 = case shown="True" w287 {
              tunnel: [w293 w296] -> w292
              tunnel: w290 -> [w293 w295]
              tunnel: w288 -> [_ w294]
              frame False {
              }
              frame True {
                n91 = invoke class="VI" method="FP.Close"(reference=w294, error in=w295) -> (error out=w296:errorcluster)  [unwired: 1 in, 2 out]
              }
            }
          }
        }
      }
      frame "---------- Macro ----------" {
        # "Do not put any code in this frame.\n(It is a separator no-op. You can make a copy of this frame to create a new Macro frame)"
      }
      frame "Macro: Initialize" {
        w302 = "Data: Initialize\nInitialize Core Data\nUI: Initialize\nUI: Front Panel State >> Open"  # Data: Initialize Initialize Core Data UI: Initialize UI: Front Panel State >> Open
        # "Initialization Macro\n(This is called once, when the VI starts)"
        n92 = call <vilib>:"Add State(s) to Queue__jki_lib_state_machine.vi"("State(s) in Front (\"\")"=w302, "State(s) in (\"\")"=w306) -> ("States Out"=w305:string)  [unwired: 13 in]
      }
      frame "Macro: Exit" {
        # "Exit Macro\n(This is called once, when the VI exits)"
        n93 = Unbundle By Name(w314) -> ("Core.Close Panel on Exit?"=w313:bool)
        n94 = Select(t="UI: Front Panel State >> Close", s=w313, f="") -> (s? t:f=w310:string)
        n95 = call <vilib>:"Add State(s) to Queue__jki_lib_state_machine.vi"("State(s) in (\"\")"=w310, "State(s) at Back (\"\")"="Data: Cleanup\nActor: Cleanup\nExit") -> ("States Out"=w308:string)  [unwired: 13 in]
        n96 = call <vilib>:"Add State(s) to Queue__jki_lib_state_machine.vi"("State(s) in Front (\"\")"=w308, "State(s) in (\"\")"=w317) -> ("States Out"=w316:string)  [unwired: 13 in]
      }
      frame "---------- New Category ----------" {
        # "Template Separator\n(You can make a copy of, or modify, this frame)"
        n97 = call <vilib>:"Add State(s) to Queue__jki_lib_state_machine.vi"("State(s) in (\"\")"=w322) -> ("States Out"=w321:string)  [unwired: 14 in]
      }
      frame "New Category: 1" {
        # "Your code here.\n(You can make a copy of, or modify, this frame)"
        n98 = call <vilib>:"Add State(s) to Queue__jki_lib_state_machine.vi"("State(s) in (\"\")"=w327) -> ("States Out"=w326:string)  [unwired: 14 in]
      }
      frame "New Category: 2" {
        # "Your code here.\n(You can make a copy of, or modify, this frame)"
        n99 = call <vilib>:"Add State(s) to Queue__jki_lib_state_machine.vi"("State(s) in (\"\")"=w332) -> ("States Out"=w331:string)  [unwired: 14 in]
      }
    }
  }
